vi "CNT Stop.vi"(10 "ChannelMask":u8, 11 "DevHandle":i32) -> (3 "function return":i32)   [LabVIEW 2010, in "usb2cnt.lvlib"]
doc: "int WINAPI CNT_Stop(int DevHandle, unsigned char ChannelMask);"
uses:
  usb2cnt.lvlib
  USB2XXX.dll
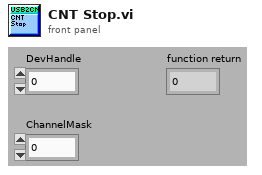
[diagram p1: front panel]
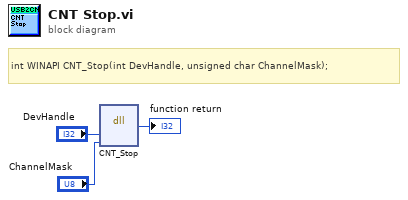
[diagram p0: block diagram]
diagram:
  # "int WINAPI CNT_Stop(int DevHandle, unsigned char ChannelMask);"
  n1 = dll-call lib="G:/OtherWork/USB2XXX_Example/trunk/Labview/PublicFiles/USB2XXX.*" fn="CNT_Stop"("DevHandle"="DevHandle", "ChannelMask"="ChannelMask") -> (→"function return":i32)  [unwired: 5 in, 2 out]
